vi "Set ICommunicate.vi"(8 "error in (no error)":errorcluster, 10 "ICommunicate":refnum<class "ICommunicate.lvclass">, 11 "NEOXID480HTA in":refnum<class "NEOXID480.lvclass">) -> (0 "error out":errorcluster, 3 "NEOXID480HTA out":refnum<class "NEOXID480.lvclass">)   [LabVIEW 2024, in "NEOXID480.lvclass"]
uses:
  NEOXID480.lvclass
  NEOXID480.lvclass/NEOXID480.ctl
  Source/Interfaces/ICommunicate/ICommunicate.lvclass
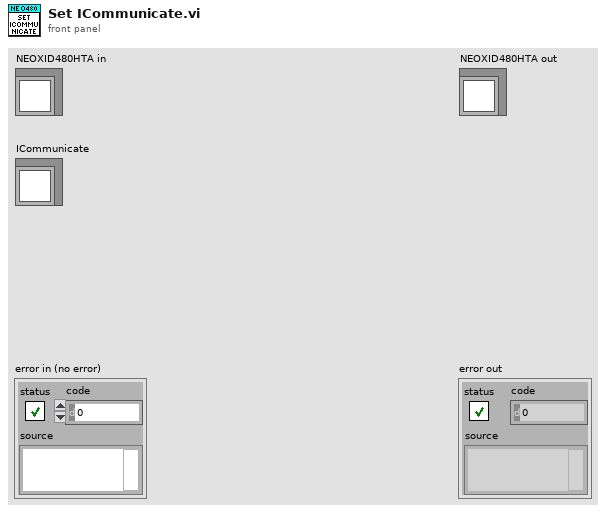
[diagram p1: front panel]
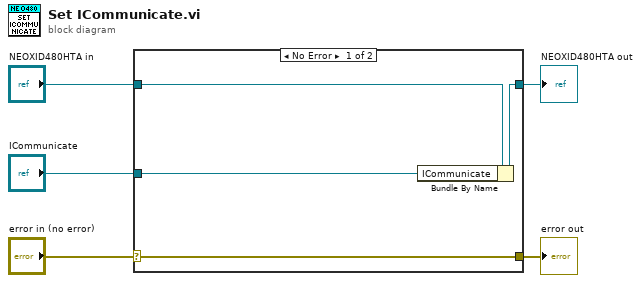
[diagram p0: block diagram]
diagram:
  n1 = case shown="No Error" "error in (no error)" {
    selector: "error in (no error)" -> [w9 w10]
    tunnel: [w9 w10] -> w4
    tunnel: [w7 w11] -> w2
    tunnel: "NEOXID480HTA in" -> [w8 w11]
    tunnel: "ICommunicate" -> [w6 _]
    frame No Error {
      n2 = Bundle By Name(cluster=w8, "ICommunicate"=w6) -> (w7:refnum<class "NEOXID480.lvclass">)
    }
    frame Error {
    }
  }
  "error out" <- w4
  "NEOXID480HTA out" <- w2
